vi "HW_Gantner_Read Buffer.vi"(0 "e.gate Configuration In":T2, 1 "InUsedChanIdx[]":i32[](array[numeric]), 2 "InUsedPhyCH[]":T1, 3 "DataBuf":refnum<queue>, 5 "CurrentT0":timestamp, 7 "Iteration":i32=1000, 9 "dt":dbl, 11 "error in":errorcluster, 12 "StartT0":timestamp) -> (4 "e.gate Configuration Out":T2, 6 "StartT0 out":timestamp, 8 "data length":i32, 15 "error out":errorcluster)   [LabVIEW 2016]
doc: "<B>AMC - Analytik & Messtechnik GmbH Chemnitz</B>\n\nLabVIEW Drivers for e.gate / e.pac series from Gantner Instruments\n\nThis VI reads a value specified by <B>Channel</B> from a device specified by <B>connection ID In</B>."
uses:
  GantnerDriver/Gantner-Instruments HighSpeedPort/e.gate Configuration.ctl
  GantnerDriver/Gantner-Instruments HighSpeedPort/e.gate Channel Data.ctl
  GantnerDriver/Gantner-Instruments HighSpeedPort/e.gate Data Type.ctl
  GantnerDriver/Gantner-Instruments HighSpeedPort/e.gate Protocol Type.ctl
  GantnerDriver/Gantner-Instruments HighSpeedPort/e.gate Module  Data.ctl
  GantnerDriver/Gantner-Instruments HighSpeedPort/e.gateHSP_DLLhandle.ctl
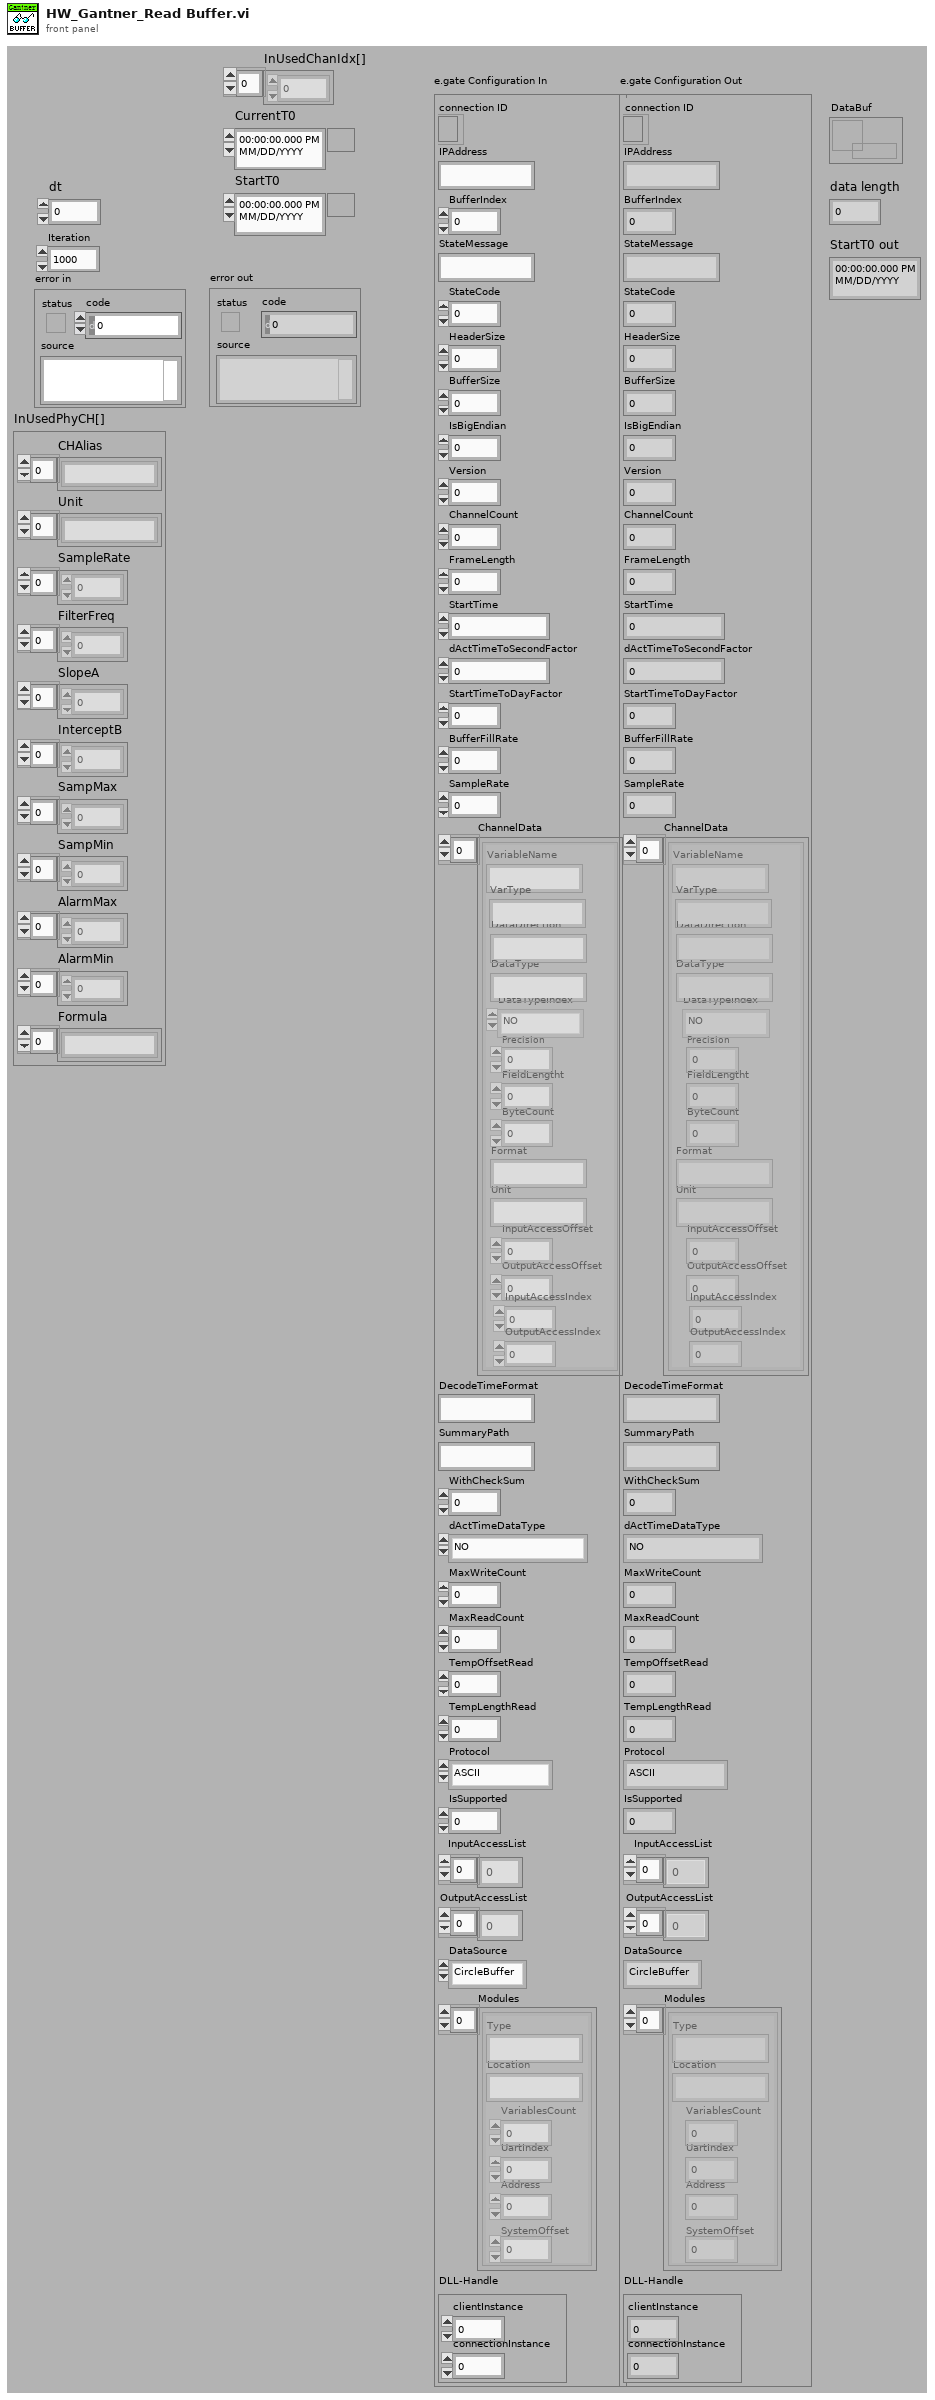
[diagram p1: front panel]
types:
  T1 = cluster{"CHAlias":string[], "Unit":string[], "SampleRate":dbl[], "FilterFreq":dbl[], "SlopeA":dbl[], "InterceptB":dbl[], "SampMax":dbl[], "SampMin":dbl[], "AlarmMax":dbl[], "AlarmMin":dbl[], "Formula":string[]}
  T2 = typedef "e.gate Configuration.ctl" = cluster{"connection ID":refnum<k5>, "IPAddress":string, "BufferIndex":i32, "StateMessage":string, "StateCode":i8, "HeaderSize":i32, "BufferSize":i32, "IsBigEndian":i32, "Version":i32, "ChannelCount":i32, "FrameLength":i32, "StartTime":dbl, "dActTimeToSecondFactor":dbl, "StartTimeToDayFactor":dbl, "BufferFillRate":dbl, "SampleRate":dbl, "ChannelData":T3[], "DecodeTimeFormat":string, "SummaryPath":string, "WithCheckSum":i32, "dActTimeDataType":T4, "MaxWriteCount":i32, "MaxReadCount":i32, "TempOffsetRead":i32, "TempLengthRead":i32, "Protocol":T5, "IsSupported":i32, "InputAccessList":i32[], "OutputAccessList":i32[], "DataSource":enum16{"CircleBuffer", "test.con Logger", "test.con Archive"}, "Modules":T6[], "DLL-Handle":T7}
  T3 = typedef "e.gate Channel Data.ctl" = cluster{"VariableName":string, "DataDirection":string, "DataType":string, "DataTypeIndex":T4, "Precision":i16, "FieldLengtht":i16, "ByteCount":i32, "Format":string, "Unit":string, "InputAccessOffset":i32, "OutputAccessOffset":i16, "InputAccessIndex":i16, "OutputAccessIndex":i16, "VarType":string}
  T4 = typedef "e.gate Data Type.ctl" = enum16{"NO", "BOOL", "SINT8", "USINT8", "SINT16", "USINT16", "SINT32", "USINT32", "FLOAT", "SET8", "SET16", "SET32", "DOUBLE", "SINT64", "USINT64", "SET64"}
  T5 = typedef "e.gate Protocol Type.ctl" = enum16{"ASCII", "HighspeedPort Online", "HighspeedPort Buffer", "eGateHighspeedPortDLL "}
  T6 = typedef "e.gate Module  Data.ctl" = cluster{"Type":string, "Location":string, "VariablesCount":i16, "UartIndex":i16, "Address":i16, "SystemOffset":i16}
  T7 = typedef "e.gateHSP_DLLhandle.ctl" = cluster{"clientInstance":i32, "connectionInstance":i32}
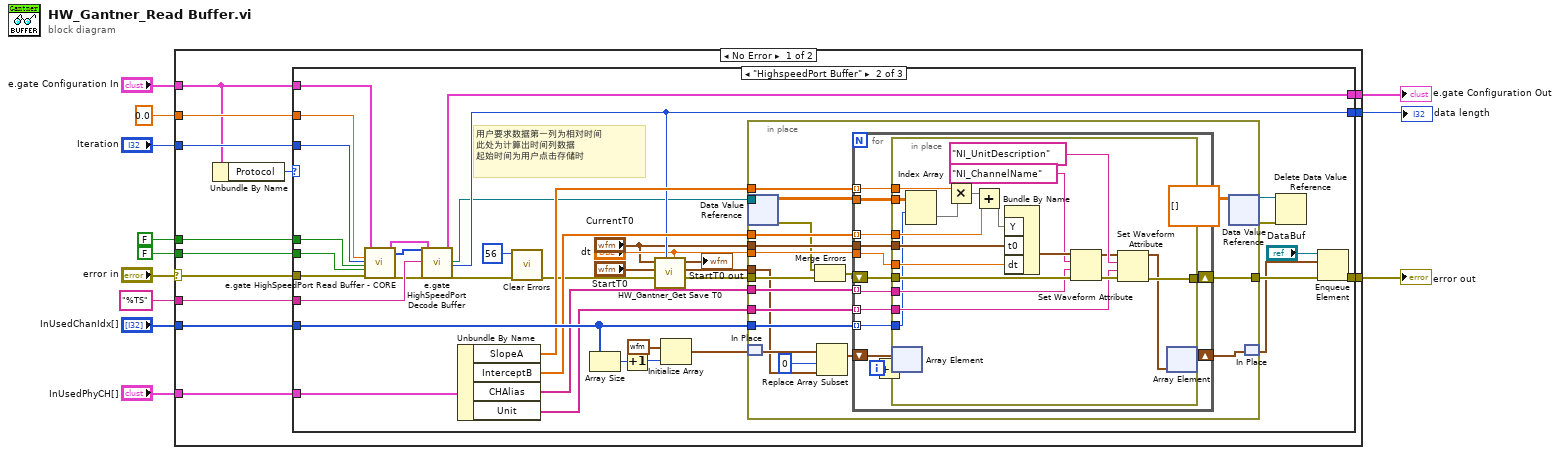
[diagram p0: block diagram]
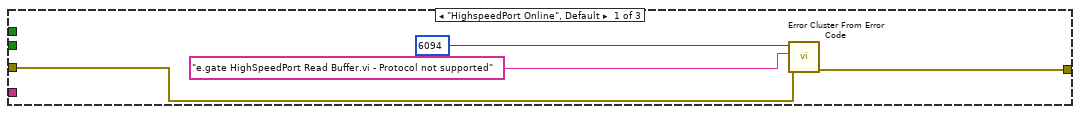
[diagram p2: hidden frame]
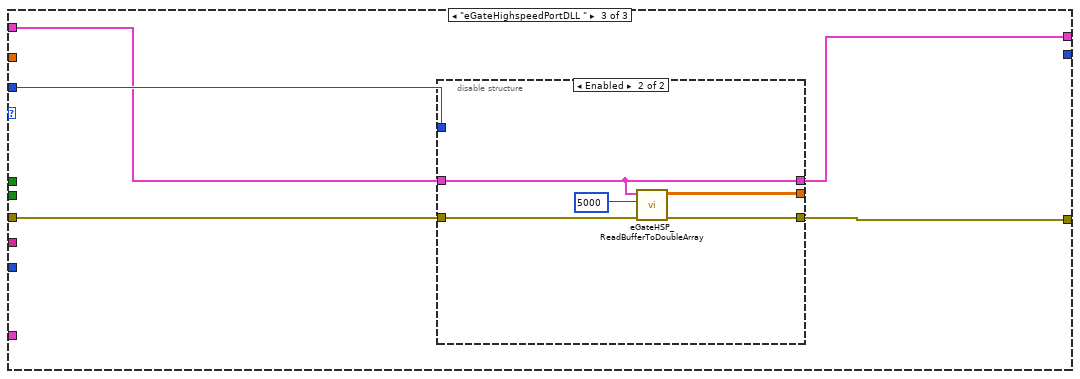
[diagram p3: hidden frame]
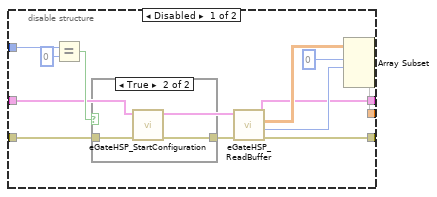
[diagram p4: hidden frame]
diagram:
  n1 = case shown="No Error" "error in" {
    selector: "error in" -> [w19 w145]
    tunnel: "e.gate Configuration In" -> [w18 w144]
    tunnel: [w25 w144] -> w10
    tunnel: [w13 w145] -> w9
    tunnel: 0.0 ("Backtime") -> [w24 _]
    tunnel: "Iteration" -> [w23 _]
    tunnel: FALSE ("force Backtime") -> [w22 _]
    tunnel: FALSE ("No Erasing") -> [w21 _]
    tunnel: "%TS" ("DecodeTimeFormat") -> [w20 _]
    tunnel: [w16 _] -> w3
    tunnel: "InUsedChanIdx[]" -> [w15 _]
    tunnel: "InUsedPhyCH[]" -> [w14 _]
    frame No Error {
      n2 = Unbundle By Name(w18) -> ("Protocol"=w17:T5)
      n3 = case shown="\"HighspeedPort Buffer\"" w17 {
        tunnel: [_ w67 w120] -> w25
        tunnel: w18 -> [_ w66 w121]
        tunnel: w24 -> [_ w63 _]
        tunnel: w23 -> [_ w62 w123]
        tunnel: w22 -> [_ w61 _]
        tunnel: w21 -> [_ w60 _]
        tunnel: w20 -> [_ w59 _]
        tunnel: w19 -> [w28 w58 w122]
        tunnel: [w27 w36 w119] -> w13
        tunnel: [_ w48 _] -> w16
        tunnel: w15 -> [_ w56 _]
        tunnel: w14 -> [_ w54 _]
        frame "HighspeedPort Online", Default {
          n4 = call <vilib>:"Error Cluster From Error Code.vi"("error in (no error)"=w28, "error message (\"\")"="e.gate HighSpeedPort Read Buffer.vi - Protocol not supported" ("error message (\"\")"), "error code (0)"=i16 6094 ("y")) -> ("error out"=w27:errorcluster)  [unwired: 1 in, 5 out]
        }
        frame "HighspeedPort Buffer" {
          # "用户要求数据第一列为相对时间\n此处为计算出时间列数据\n起始时间为用户点击存储时"
          n5 = call "e.gate HighSpeedPort Read Buffer - CORE.vi"("Backtime"=w63, "Iteration"=w62, "force Backtime"=w61, "No Erasing"=w60, "error in (no error)"=w58, "Configuration in"=w66) -> ("Configuration out"=w65:T2, "data array (binary)"=w64:u8[], "error out"=w57:errorcluster)  [unwired: 19 out]
          n6 = call "e.gate HighSpeedPort Decode Buffer.vi"("Data in (binary)"=w64, "DecodeTimeFormat"=w59, "error in"=w57, "Configuration  in"=w65) -> ("Configuration out"=w67:T2, "data value reference"=w32:refnum<data-value>, "data length"=w48:i32, "error out"=w55:errorcluster)  [unwired: 20 out]
          n7 = Unbundle By Name(w54) -> ("SlopeA"=w50:dbl[], "InterceptB"=w51:dbl[], "CHAlias"=w53:string[], "Unit"=w52:string[])
          n8 = call <vilib>:"Clear Errors.vi"("error in (no error)"=w55, "specific error code to clear (0: all)"=56) -> ("error out"=w45:errorcluster)  [unwired: 4 in, 1 out]
          n9 = Array Size(array=w56) -> (size(s)=w41:i32)
          n10 = Increment(x=w41) -> (x+1=w38:i32)
          n11 = call "HW_Gantner_Get Save T0.vi"("dt"="dt", "data length"=w48, "error in"=w45, "StartT0"="StartT0", "T0 in"="CurrentT0") -> ("error out"=w43:errorcluster, "TimeCh data"=w39:waveform(dbl), "T0 out"=→"StartT0 out":timestamp)  [unwired: 4 in]
          n12 = Initialize Array(waveform(dbl) {"t0"=timestamp(0 s since 1904-01-01), "dt"=1.0, "Y"=[]} ("output waveform"), w38) -> (w40:waveform(dbl)[])
          n13 = in-place {
            in-place-border: w53 -> [w85]
            in-place-border: w52 -> [w84]
            in-place-border: w51 -> [w83]
            in-place-border: w50 -> [w82]
            in-place-border: w32 -> [_]
            in-place-border: [w81] -> w37
            in-place-border: "dt" -> [w80]
            in-place-border: "CurrentT0" -> [w79]
            in-place-border: w43 -> [w78]
            in-place-border: w56 -> [w77]
            in-place-border: w39 -> [w73]
            n14 = in-place-dvr #1(w32) -> (w71:dbl[][], w68:errorcluster)
            n15 = in-place-match #2(w40) -> (w75:waveform(dbl)[])
            n16 = Merge Errors(w68, w78) -> (w69:errorcluster)
            n17 = Replace Array Subset(array=w75, new element=w73, index=0) -> (w76:waveform(dbl)[])
            n18 = for {
              tunnel: w80 -> [w99]
              tunnel: w79 -> [w98]
              shift-right: [w96] -> w81
              shift-left: w69 -> [w97]
              tunnel: w85 -> [w95] mode=indexing
              tunnel: w84 -> [w94] mode=indexing
              tunnel: w82 -> [w93] mode=indexing
              tunnel: w83 -> [w92] mode=indexing
              tunnel: w71 -> [w91]
              tunnel: w77 -> [w90] mode=indexing
              shift-right: [w87] -> w72
              shift-left: w76 -> [w89]
              i -> [w88]
              n19 = Increment(x=w88) -> (x+1=w86:i32)
              n20 = in-place {
                in-place-border: w99 -> [w118]
                in-place-border: w98 -> [w117]
                in-place-border: w97 -> [w114]
                in-place-border: [w112] -> w96
                in-place-border: w95 -> [w109]
                in-place-border: w94 -> [w108]
                in-place-border: w93 -> [w106]
                in-place-border: w92 -> [w105]
                in-place-border: w91 -> [w103]
                in-place-border: w90 -> [w101]
                n21 = in-place-array #3(w89, w86) -> ()  [unwired: 1 out]
                n22 = Index Array(array=w103, index (row)=w101) -> (element=w102:dbl[])  [unwired: 1 in]
                n23 = Multiply(x=w106, y=w102) -> (x*y=w107:dbl[])
                n24 = Add(x=w107, y=w105) -> (x+y=w104:dbl[])
                n25 = Bundle By Name("Y"=w104, "t0"=w117, "dt"=w118) -> (w116:waveform(dbl))  [unwired: 1 in]
                n26 = Set Waveform Attribute(4:w114, 5:w109, 6:"NI_ChannelName" ("名称"), 7:w116) -> (0:w113:errorcluster, 3:w110:waveform(dbl))  [unwired: 1 out]
                n27 = Set Waveform Attribute(4:w113, 5:w108, 6:"NI_UnitDescription" ("名称"), 7:w110) -> (0:w112:errorcluster, 3:w100:waveform(dbl))  [unwired: 1 out]
                n28 = in-place-array #3(w100) -> (w87:waveform(dbl)[])  [unwired: 1 out]
              }
            }
            n29 = in-place-dvr #1(dbl[][] [] ("data value")) -> (w30:refnum<data-value>, w31:errorcluster)
            n30 = in-place-match #2(w72) -> (w35:waveform(dbl)[])
          }
          n31 = Delete Data Value Reference(data value reference=w30, error in=w31) -> ()  [unwired: 2 out]
          n32 = Enqueue Element(queue="DataBuf", element=w35, error in (no error)=w37) -> (error out=w36:errorcluster)  [unwired: 1 in, 2 out]
        }
        frame "eGateHighspeedPortDLL " {
          n33 = disable-structure shown="Enabled" {
            disable-tunnel: w123 -> [w135 _]
            disable-tunnel: w122 -> [w132 w139]
            disable-tunnel: w121 -> [w130 w140]
            disable-tunnel: [w126 w141] -> _
            disable-tunnel: [w125 w140] -> w120
            disable-tunnel: [w124 w142] -> w119
            frame Disabled {
              n34 = Equal?(x=w135, y=0) -> (x = y?=w133:bool)
              n35 = case shown="True" w133 {
                tunnel: w132 -> [w136 w138]
                tunnel: [w136 w137] -> w131
                frame False {
                }
                frame True {
                  n36 = call "eGateHSP_StartConfiguration.vi"("Fehler (Eingang, kein Fehler)"=w138) -> ("Fehler (Ausgang)"=w137:errorcluster)  [unwired: 10 in]
                }
              }
              n37 = call "eGateHSP_ReadBuffer.vi"("Fehler (Eingang, kein Fehler)"=w131, "e.gate Configuration"=w130) -> ("Fehler (Ausgang)"=w124:errorcluster, "number of Frames"=w128:i32, "Array"=w129:dbl[][], "e.gate Configuration 2"=w125:T2)  [unwired: 4 in]
              n38 = Array Subset(array=w129, index (row)=0 ("Index"), length (row)=w128) -> (w126:dbl[][])  [unwired: 2 in]
            }
            frame Enabled {
              n39 = call "eGateHSP_ReadBufferToDoubleArray.vi"("Fehler (Eingang, kein Fehler)"=w139, "NumberOfFrames"=5000, "e.gate Configuration"=w140) -> ("Fehler (Ausgang)"=w142:errorcluster, "Array (Ausgang)"=w141:dbl[][])  [unwired: 7 in]
            }
          }
        }
      }
    }
    frame Error {
    }
  }
  "error out" <- w9
  "e.gate Configuration Out" <- w10
  "data length" <- w3
